vi "Read.vi"(8 "error in":errorcluster, 11 "CANopen Master in":refnum<class "CANopen Master.lvclass">) -> (0 "error out":errorcluster, 1 "Empty?":bool, 2 "CANopen Message out":refnum<class "CANopen Response Message.lvclass">, 3 "CANopen Master out":refnum<class "CANopen Master.lvclass">)   [LabVIEW 2024, in "CANopen Master.lvclass"]
uses:
  CANopen Master.lvclass
  CANopen Master.lvclass/CANopen Master.ctl
  CANopen Response/CANopen Response Message.lvclass
  source/CANopen Message/CANopen Message.lvclass
  HAL/Source/Interfaces/IMessage/IMessage.lvclass
  HAL/Source/Interfaces/ICommunicate/ICommunicate.lvclass
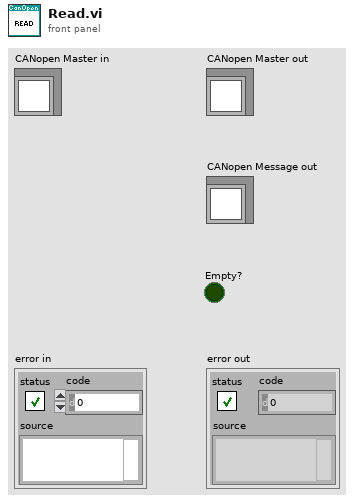
[diagram p1: front panel]
types:
  T1 = map{string, refnum<class "ICommunicate.lvclass">}
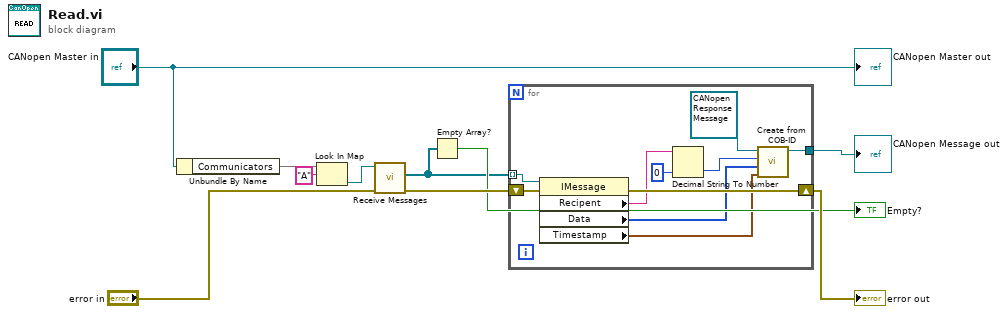
[diagram p0: block diagram]
diagram:
  n1 = Unbundle By Name("CANopen Master in") -> ("Communicators"=w3:T1)
  n2 = Look In Map(map=w3, key="A") -> (value=w1:refnum<class "ICommunicate.lvclass">)  [unwired: 1 in, 1 out]
  n3 = call-dynamic "Receive Messages.vi"("error in"="error in", "ICommunicate in"=w1) -> ("error out"=w9:errorcluster, "Messages"=w4:refnum<class "IMessage.lvclass">[])  [unwired: 7 in, 1 out]
  n4 = Empty Array?(array=w4) -> (empty?=→"Empty?":bool)
  n5 = for {
    tunnel: [w18] -> w6
    tunnel: w4 -> [w16] mode=indexing
    shift-right: [w19] -> w8
    shift-left: w9 -> [w20]
    n6 = property class="IMessage"(reference=w16, error in=w20) -> (error out=w19:errorcluster, "Recipent"=w14:string, "Data"=w15:u8[], "Timestamp"=w11:timestamp)  [unwired: 1 out]
    n7 = Decimal String To Number(string=w14, default (0L)=u32 0) -> (number=w13:u32)  [unwired: 1 in, 1 out]
    n8 = call "Create from COB-ID.vi"("Timestamp"=w11, "Data"=w15, "COB-ID"=w13, 11:refnum<class "CANopen Response Message.lvclass"> refnum ("CANopen Master.lvlib:CANopen Request.lvclass")) -> ("CANopen Message out"=w18:refnum<class "CANopen Message.lvclass">)  [unwired: 7 in]
  }
  "error out" <- w8
  "CANopen Message out" <- w6
  "CANopen Master out" <- "CANopen Master in"
